vi "Principal.vi"() -> ()   [LabVIEW 2014]
panel:
  in  "Temperatura °C":dbl
  out "Grados":string
  out "Thermometer":dbl(slide) scale=0.0..1000.0
  in  "Enum":enum16{"°C to °F", "°C to °K", "°C to °R"}(ring)
  in  "stop":bool
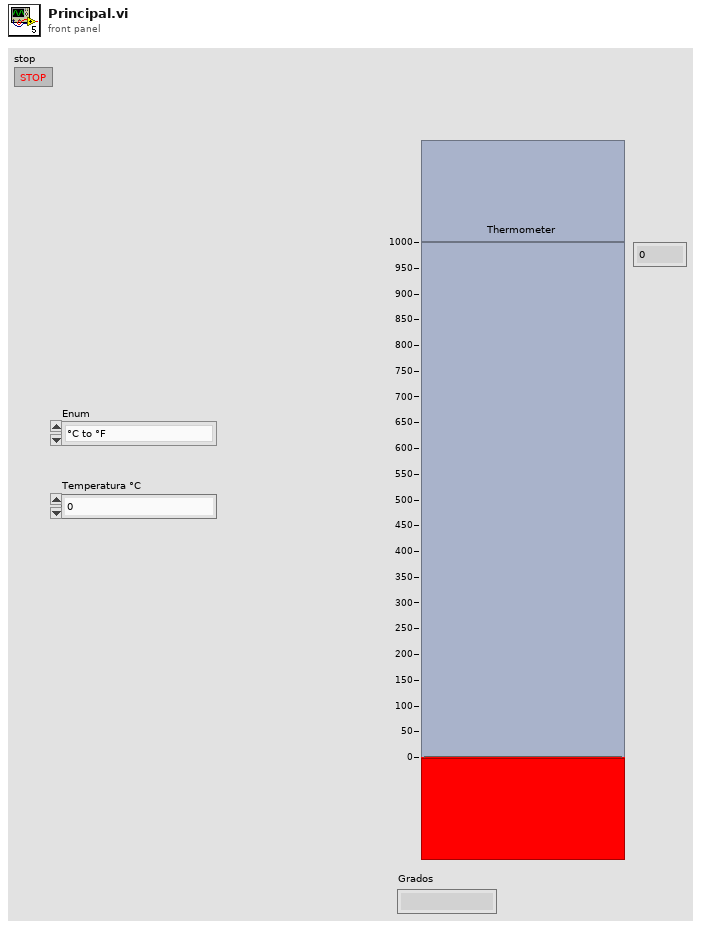
[diagram p1: front panel]
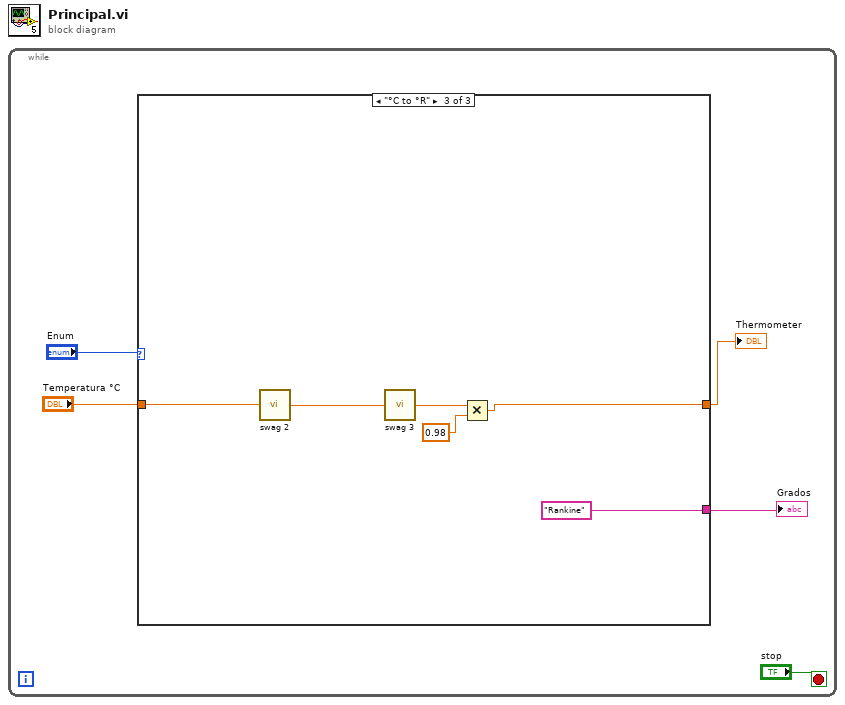
[diagram p0: block diagram]
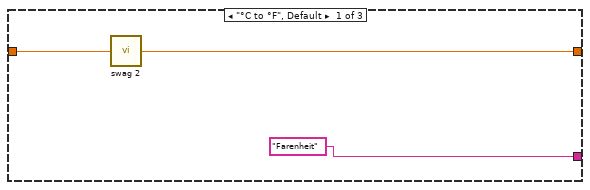
[diagram p2: hidden frame]
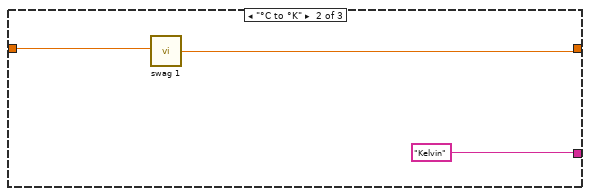
[diagram p3: hidden frame]
diagram:
  n1 = while {
    stop <- "stop" stop-if-true
    n2 = case shown="\"°C to °R\"" "Enum" {
      tunnel: "Temperatura °C" -> [w8 w11 w17]
      tunnel: [w7 w10 w12] -> w2
      tunnel: ["Farenheit" "Kelvin" "Rankine"] -> w1
      frame "°C to °F", Default {
        n3 = call "swag 2.vi"("Numeric"=w8) -> ("°Farenheit"=w7:dbl)
      }
      frame "°C to °K" {
        n4 = call "swag 1.vi"("Temperatura °C"=w11) -> ("°Kelvin"=w10:dbl)
      }
      frame "°C to °R" {
        n5 = call "swag 2.vi"("Numeric"=w17) -> ("°Farenheit"=w16:dbl)
        n6 = call "swag 3.vi"("°Farenheit"=w16) -> ("Rankine"=w14:dbl)
        n7 = Multiply(x=w14, y=0.98) -> (x*y=w12:dbl)
      }
    }
    "Grados" <- w1
    "Thermometer" <- w2
  }
